vi "Flasher.vi"() -> ()   [LabVIEW 2017]
uses:
  GlobalFlash.vi
panel:
  out "?":bool
  out "?":bool
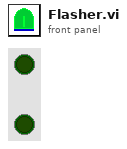
[diagram p1: front panel]
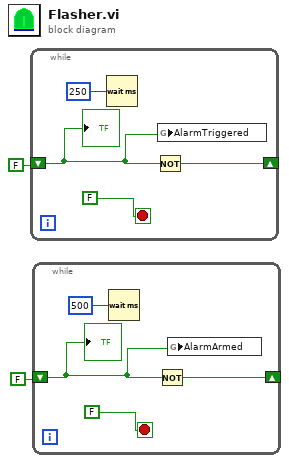
[diagram p0: block diagram]
diagram:
  n1 = while {
    shift-right: [w5] -> _
    shift-left: FALSE -> [w3]
    stop <- FALSE stop-if-true
    n2 = Wait (ms)(milliseconds to wait=250) -> ()  [unwired: 1 out]
    n3 = Not(x=w3) -> (.not. x?=w5:bool)
    n4 = global write "GlobalFlash.vi" "AlarmTriggered"(w3) -> ()
    "?" <- w3
  }
  n5 = while {
    shift-right: [w9] -> _
    shift-left: FALSE -> [w7]
    stop <- FALSE stop-if-true
    n6 = Wait (ms)(milliseconds to wait=500) -> ()  [unwired: 1 out]
    n7 = Not(x=w7) -> (.not. x?=w9:bool)
    n8 = global write "GlobalFlash.vi" "AlarmArmed"(w7) -> ()
    "?" <- w7
  }
